vi "Get Attribut Caméra.vi"(8 "entrée d'erreur (pas d'erreur)":errorcluster, 9 "Shutter Caméra":refnum<vi>, 10 "Gain Caméra":refnum<vi>, 11 "Data Cam Processing":T1 {"sigma X" format="%0.2f"; "mean X" format="%0.2f"; "mean Y" format="%0.2f"; "sigma Y" format="%0.2f"; "Shutter (us)" scale=22.0..10000000.0; "Gain Caméra" scale=0.0..1023.0}) -> (0 "sortie d'erreur":errorcluster, 3 "Data Cam Processing out":T1 {"sigma X" format="%0.2f"; "mean X" format="%0.2f"; "mean Y" format="%0.2f"; "sigma Y" format="%0.2f"; "Shutter (us)" scale=22.0..10000000.0; "Gain Caméra" scale=0.0..1023.0})   [LabVIEW 2026]
uses:
  Data-Processing.ctl
  <vilib>/Serenial/G Industrial Camera/g_industrial_cam/Camera/Camera.lvclass
  <vilib>/Serenial/G Industrial Camera/g_industrial_cam/Buffer/Buffer.lvclass
  <vilib>/picture/picture.llb/imagedata.ctl
  <vilib>/Serenial/G Industrial Camera/g_industrial_cam/Camera/Camera.lvclass/Camera.ctl
  <vilib>/Serenial/G Industrial Camera/g_industrial_cam/Camera/GetSetGain.vi
  <vilib>/Serenial/G Industrial Camera/g_industrial_cam/Camera/GetSetExposureTime.vi
  <vilib>/Serenial/G Industrial Camera/g_industrial_cam/Camera/Check Not Disconnected.vi
  <vilib>/Utility/error.llb/Error Cluster From Error Code.vi
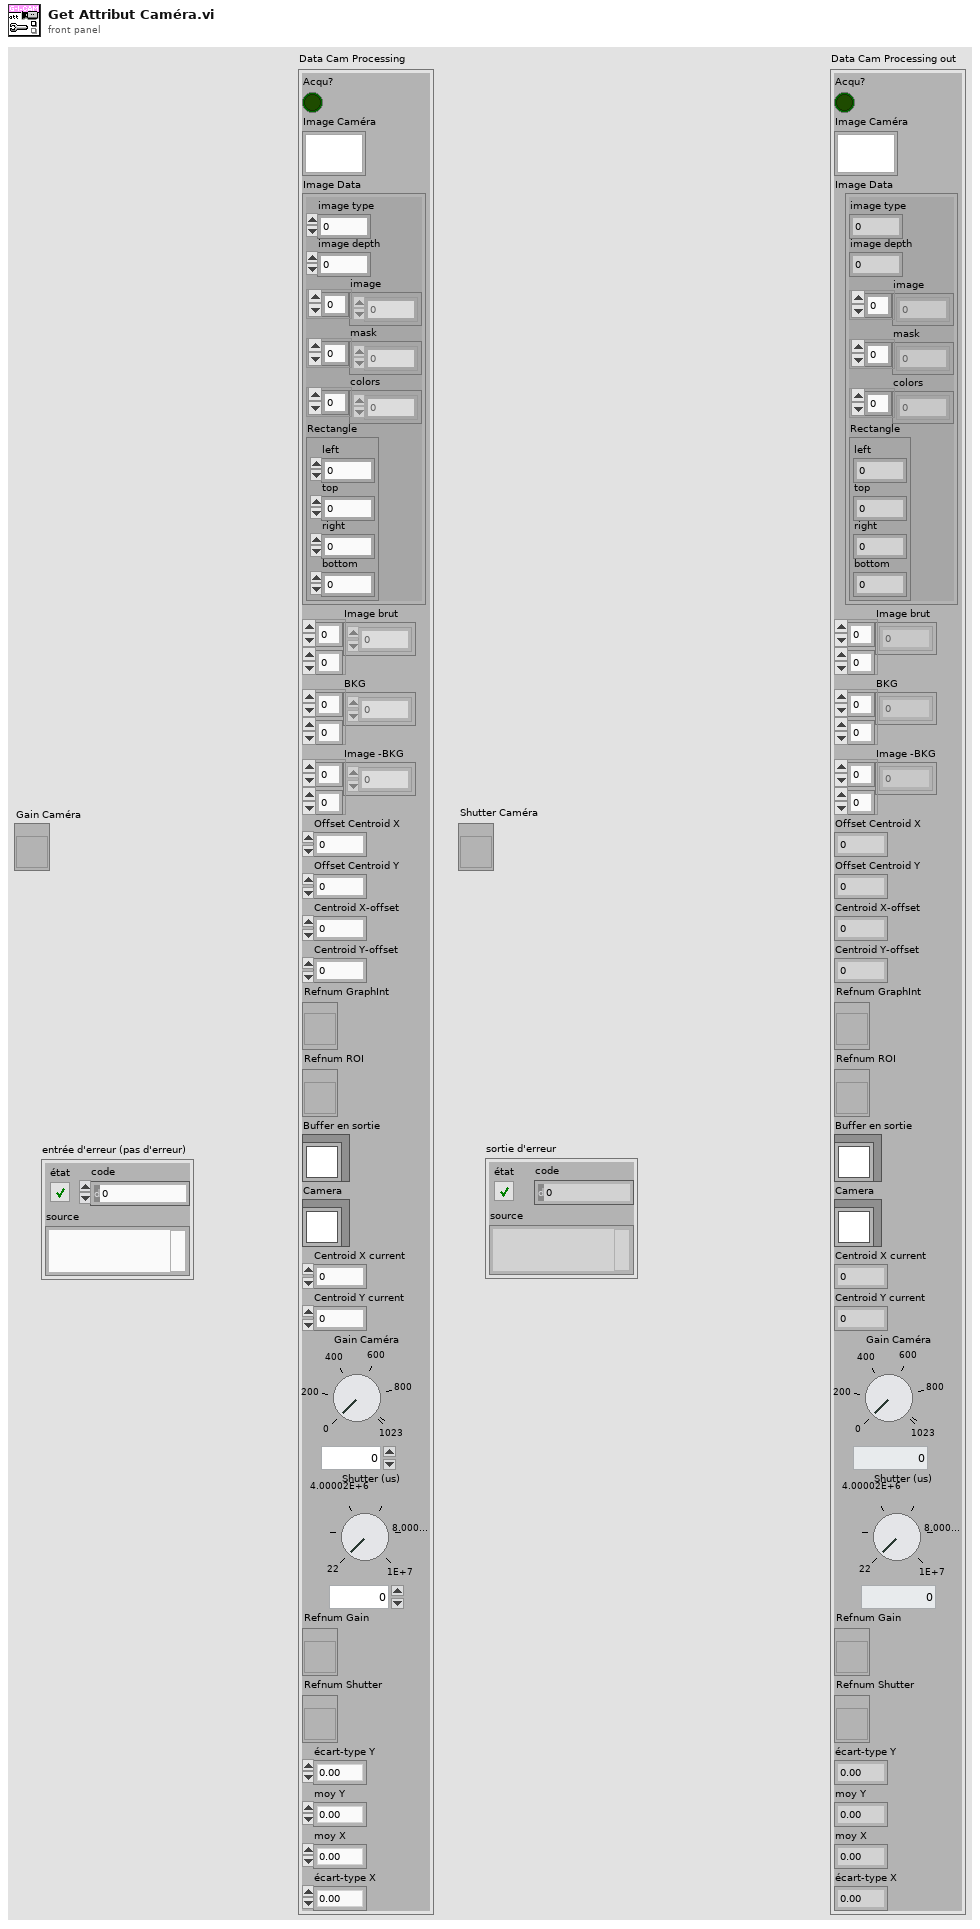
[diagram p1: front panel]
types:
  T1 = typedef "Data-Processing.ctl" = cluster{"Acqu?":bool, "Image Caméra":picture, "Image Data":T2, "Image brut":i16[][], "BKG":i16[][], "Image -BKG":i16[][], "Offset Centroid X":dbl, "Offset Centroid Y":dbl, "Centroid X-offset":dbl, "Centroid Y-offset":dbl, "Refnum GraphInt":refnum<vi>, "Refnum ROI":refnum<vi>, "Buffer en sortie":refnum<class "Buffer.lvclass">, "Camera":refnum<class "Camera.lvclass">, "Centroid X current":dbl, "Centroid Y current":dbl, "Gain Caméra":i32, "Shutter (us)":dbl, "Refnum Gain":refnum<vi>, "Refnum Shutter":refnum<vi>, "sigma Y":dbl, "mean Y":dbl, "mean X":dbl, "sigma X":dbl}
  T2 = typedef "imagedata.ctl" = cluster{"image type":i32, "image depth":i32, "image":u8[], "mask":u8[], "colors":u32[], "Rectangle":cluster{"left":i16, "top":i16, "right":i16, "bottom":i16}}
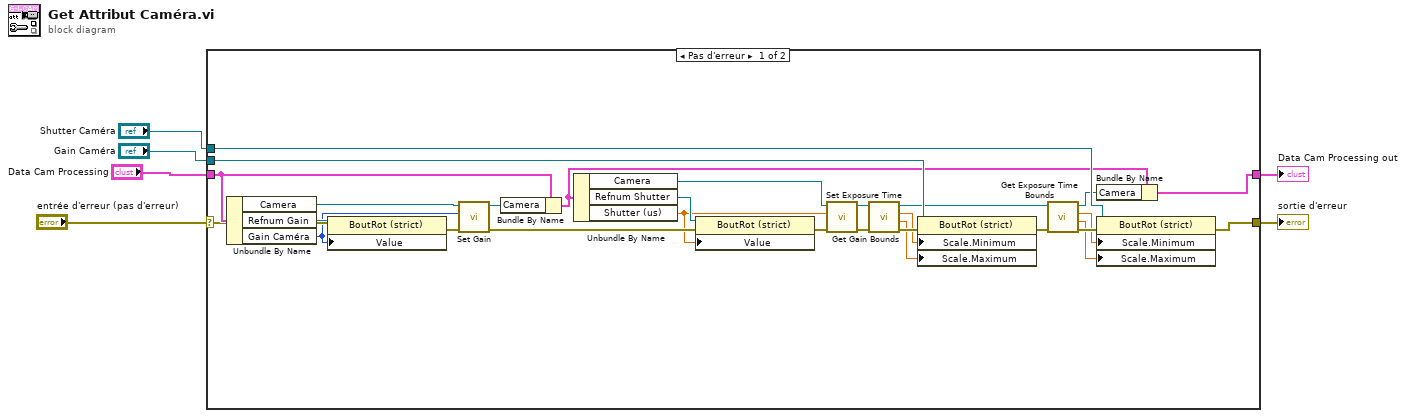
[diagram p0: block diagram]
diagram:
  n1 = case shown="Pas d'erreur" "entrée d'erreur (pas d'erreur)" {
    selector: "entrée d'erreur (pas d'erreur)" -> [w15 w36]
    tunnel: "Gain Caméra" -> [w34 _]
    tunnel: [w28 w36] -> w5
    tunnel: "Shutter Caméra" -> [w26 _]
    tunnel: [w11 w35] -> w2
    tunnel: "Data Cam Processing" -> [w22 w35]
    frame No Error {
      n2 = Unbundle By Name(w22) -> ("Camera"=w17:refnum<class "Camera.lvclass">, "Refnum Gain"=w23:refnum<vi>, "Gain Caméra"=w14:i32)
      n3 = property class="BoutRot (strict)"(reference=w23, error in=w15, "Value"=w14) -> (error out=w19:errorcluster)  [unwired: 1 out]
      n4 = call <vilib>:"Set Gain.vi"("error in (no error)"=w19, "Gain"=w14, "Camera in"=w17) -> ("error out"=w18:errorcluster, "Camera"=w16:refnum<class "Camera.lvclass">)  [unwired: 7 in]
      n5 = Bundle By Name(cluster=w22, "Camera"=w16) -> (w20:T1)
      n6 = Unbundle By Name(w20) -> ("Camera"=w13:refnum<class "Camera.lvclass">, "Refnum Shutter"=w21:refnum<vi>, "Shutter (us)"=w8:dbl)
      n7 = property class="BoutRot (strict)"(reference=w21, error in=w18, "Value"=w8) -> (error out=w9:errorcluster)  [unwired: 1 out]
      n8 = call <vilib>:"Set Exposure Time.vi"("error in (no error)"=w9, "Time (us)"=w8, "Camera in"=w13) -> ("error out"=w7:errorcluster, "Camera"=w12:refnum<class "Camera.lvclass">)  [unwired: 7 in]
      n9 = call <vilib>:"Get Gain Bounds.vi"("error in (no error)"=w7, "Camera in"=w12) -> ("error out"=w33:errorcluster, "Max"=w32:dbl, "Min"=w31:dbl, "Camera"=w27:refnum<class "Camera.lvclass">)  [unwired: 6 in]
      n10 = property class="BoutRot (strict)"(reference=w34, error in=w33, "Scale.Minimum"=w31, "Scale.Maximum"=w32) -> (error out=w30:errorcluster)  [unwired: 1 out]
      n11 = call <vilib>:"Get Exposure Time Bounds.vi"("error in (no error)"=w30, "Camera in"=w27) -> ("error out"=w29:errorcluster, "Max (us)"=w24:dbl, "Min (us)"=w25:dbl, "Camera"=w10:refnum<class "Camera.lvclass">)  [unwired: 6 in]
      n12 = Bundle By Name(cluster=w20, "Camera"=w10) -> (w11:T1)
      n13 = property class="BoutRot (strict)"(reference=w26, error in=w29, "Scale.Minimum"=w25, "Scale.Maximum"=w24) -> (error out=w28:errorcluster)  [unwired: 1 out]
    }
    frame Error {
    }
  }
  "sortie d'erreur" <- w5
  "Data Cam Processing out" <- w2
